vi "capt.vi"(6 "Graph in":cluster{dbl[], dbl[]}, 7 "Index":i32=250, 8 "error in":errorcluster, 9 "Length":i32=250, 11 "ON":bool) -> (0 "error out":errorcluster, 2 "Values":cluster{dbl[], dbl[]})   [LabVIEW 2012]
panel:
  in  "Address":u8=250
  in  "Channel":enum16{"CH0", "P1", "P2", "T", "TOB1", "TOB2"}(ring)=enum."P1"
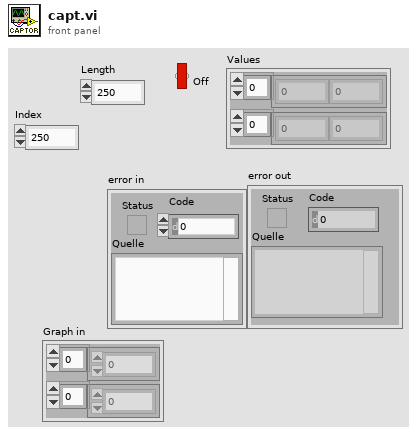
[diagram p1: front panel]
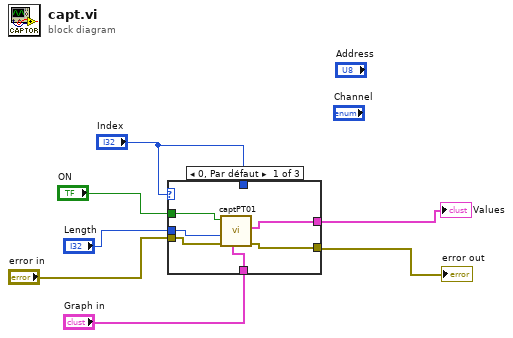
[diagram p0: block diagram]
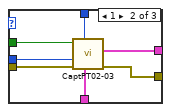
[diagram p2: hidden frame]
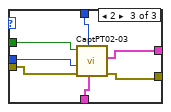
[diagram p3: hidden frame]
diagram:
  n1 = case shown="0, Par défaut" "Index" {
    tunnel: "Index" -> [_ w20 w27]
    tunnel: "ON" -> [w9 w19 w21]
    tunnel: "error in" -> [w12 w18 w23]
    tunnel: "Graph in" -> [w11 w17 w24]
    tunnel: "Length" -> [w8 w16 w22]
    tunnel: [w13 w15 w25] -> w3
    tunnel: [w10 w14 w26] -> w2
    frame 0, Default {
      n2 = call "captPT01.vi"("Graph in 2"=w11, "error in"=w12, "Length 2"=w8, "ON 2"=w9) -> ("error out 2"=w13:errorcluster, "Values 2"=w10:cluster{dbl[], dbl[]})  [unwired: 6 in]
    }
    frame 1 {
      n3 = call "CaptPT02-03.vi"("Graph in 2"=w17, "Index"=w20, "error in"=w18, "Length 2"=w16, "ON 2"=w19) -> ("error out"=w15:errorcluster, "Values 2"=w14:cluster{dbl[], dbl[]})  [unwired: 5 in]
    }
    frame 2 {
      n4 = call "CaptPT02-03.vi"("Graph in 2"=w24, "Index"=w27, "error in"=w23, "Length 2"=w22, "ON 2"=w21) -> ("error out"=w25:errorcluster, "Values 2"=w26:cluster{dbl[], dbl[]})  [unwired: 5 in]
    }
  }
  "error out" <- w3
  "Values" <- w2
